vi "Real to Norm Coordinate.vi"(5 "Zoom":dbl, 7 "FrameSize":dbl, 9 "Y":dbl, 11 "X":dbl) -> (1 "Norm. Y":dbl, 3 "Norm. X":dbl)   [LabVIEW 2017]
panel:
  out "Norm.X (Formula)":dbl
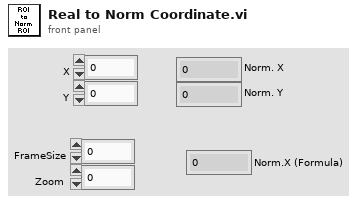
[diagram p1: front panel]
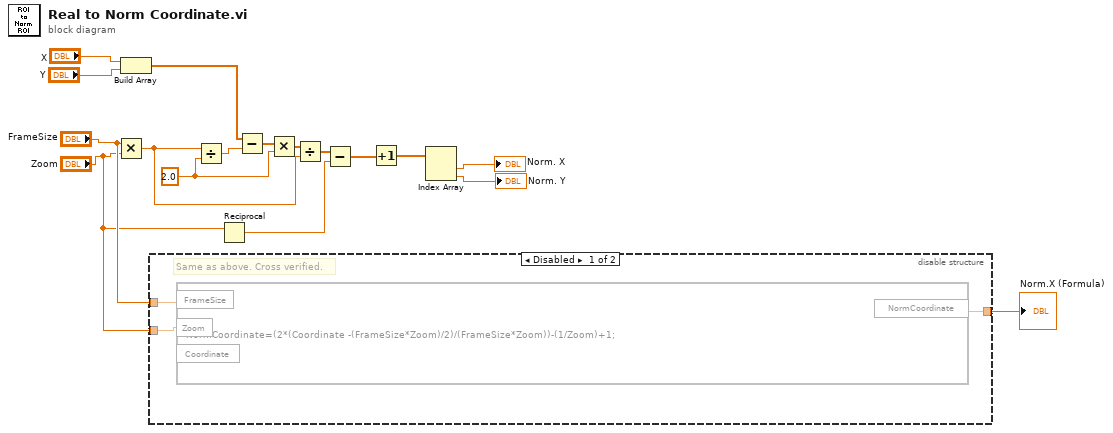
[diagram p0: block diagram]
diagram:
  w15 = 2.0 ("y")
  n1 = Multiply(x="FrameSize", y="Zoom") -> (x*y=w13:dbl)
  n2 = Build Array("X", "Y") -> (w5:dbl[])
  n3 = disable-structure shown="Disabled" {
    disable-tunnel: "FrameSize" -> [w20 _]
    disable-tunnel: "Zoom" -> [w19 _]
    disable-tunnel: [w18 _] -> w6
    frame Disabled {
      # "Same as above. Cross verified."
      n4 = formula code="NormCoordinate=(2*(Coordinate -(FrameSize*Zoom)/2)/(FrameSize*Zoom))-(1/Zoom)+1;"("FrameSize"=w20, "Zoom"=w19) -> ("NormCoordinate"=w18:dbl)  [unwired: 1 in]
    }
    frame Enabled {
    }
  }
  "Norm.X (Formula)" <- w6
  n5 = Divide(x=w13, y=w15) -> (x/y=w14:dbl)
  n6 = Reciprocal(x="Zoom") -> (1/x=w11:dbl)
  n7 = Subtract(x=w5, y=w14) -> (x-y=w16:dbl[])
  n8 = Multiply(x=w16, y=w15) -> (x*y=w17:dbl[])
  n9 = Divide(x=w17, y=w13) -> (x/y=w10:dbl[])
  n10 = Subtract(x=w10, y=w11) -> (x-y=w12:dbl[])
  n11 = Increment(x=w12) -> (x+1=w3:dbl[])
  n12 = Index Array(array=w3) -> (element #1=→"Norm. X":dbl, element #2=→"Norm. Y":dbl)  [unwired: 2 in]
